vi "Check Path for Output.vi"(8 "error in (no error)":errorcluster, 10 "Path":path) -> (0 "error out":errorcluster)   [LabVIEW 2017, in "WebServiceImporter.lvlib" / "Main Panel.lvlib" / "Input Info.lvlib"]
uses:
  <vilib>/Platform/WebService/Main Panel/Pages/Input Info/Input Info.lvlib
  <vilib>/Platform/WebService/Error Handling/Error/Error Number.ctl
  <vilib>/Platform/WebService/Error Handling/Error Handling.lvlib
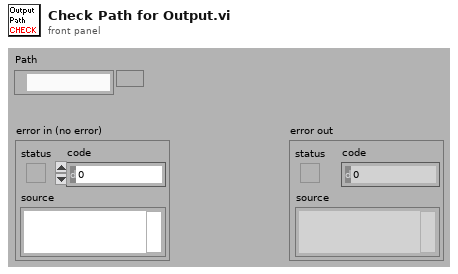
[diagram p1: front panel]
types:
  T1 = enum16{"open", "replace", "create", "open or create", "replace or create", "replace or create with confirmation"}
  T2 = typedef "WebServiceImporter.lvlib/Error Handling.lvlib/Error Number.ctl" = u16
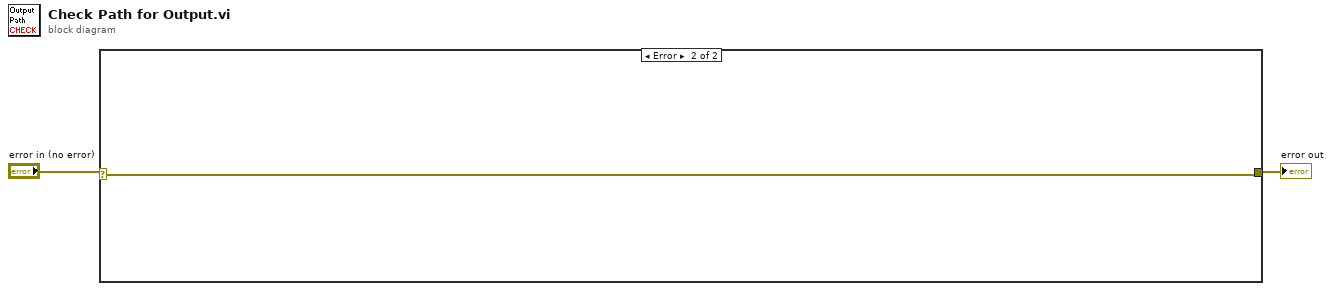
[diagram p0: block diagram]
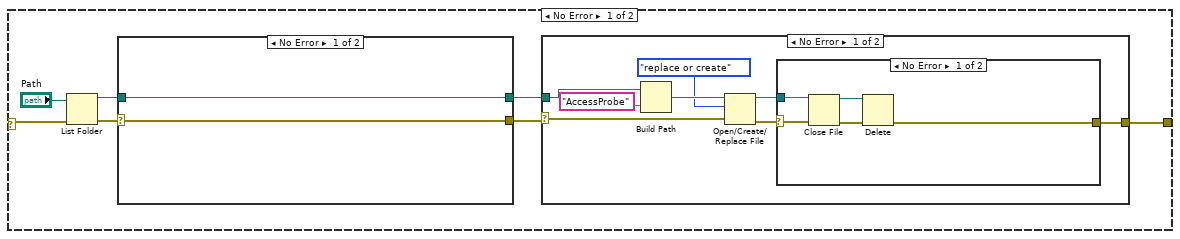
[diagram p2: hidden frame]
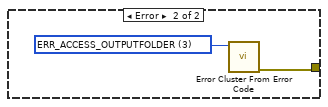
[diagram p3: hidden frame]
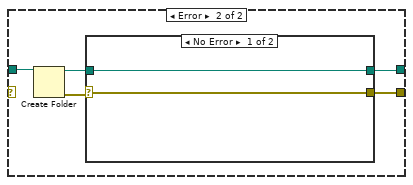
[diagram p5: hidden frame]
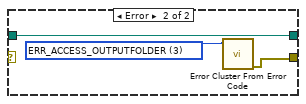
[diagram p6: hidden frame]
diagram:
  n1 = case shown="Error" "error in (no error)" {
    selector: "error in (no error)" -> [w3 w38]
    tunnel: [w5 w38] -> w2
    frame No Error {
      n2 = List Folder(path="Path", error in=w3) -> (path out=w8:path, error out=w7:errorcluster)  [unwired: 2 in, 2 out]
      n3 = case shown="No Error" w7 {
        selector: w7 -> [w27 _]
        tunnel: w8 -> [w26 w32]
        tunnel: [w27 w30] -> w6
        tunnel: [w26 w28] -> w4
        frame No Error {
        }
        frame Error {
          n4 = Create Folder(path (use dialog)=w32) -> (created path=w29:path, error out=w31:errorcluster)  [unwired: 2 in, 1 out]
          n5 = case shown="No Error" w31 {
            selector: w31 -> [w34 _]
            tunnel: [w34 w35] -> w30
            tunnel: w29 -> [w33 w37]
            tunnel: [w33 w37] -> w28
            frame No Error {
            }
            frame Error {
              w36 = T2 3 items=["No Error", "ERR_INVALID_WSDL", "ERR_CREATE_PROXYDLL", "ERR_ACCESS_OUTPUTFOLDER"] ("Error Number")
              n6 = call <vilib>:"Error Cluster From Error Code.vi"("error code (0)"=w36) -> ("error out"=w35:errorcluster)  [unwired: 8 in]
            }
          }
        }
      }
      n7 = case shown="No Error" w6 {
        selector: w6 -> [w13 w25]
        tunnel: [w10 w25] -> w5
        tunnel: w4 -> [w17 _]
        frame No Error {
          n8 = Build Path(base path=w17, name or relative path="AccessProbe") -> (appended path=w15:path)
          n9 = Open/Create/Replace File(file path (use dialog)=w15, error in=w13, operation (0:open)=T1."replace or create") -> (refnum out=w11:refnum<file>, error out=w12:errorcluster)  [unwired: 3 in, 1 out]
          n10 = case shown="No Error" w12 {
            selector: w12 -> [w22 _]
            tunnel: w11 -> [w21 _]
            tunnel: [w18 w23] -> w10
            frame No Error {
              n11 = Close File(refnum=w21, error in=w22) -> (path=w20:path, error out=w19:errorcluster)
              n12 = Delete(path (use dialog)=w20, error in=w19) -> (error out=w18:errorcluster)  [unwired: 3 in, 2 out]
            }
            frame Error {
              w24 = T2 3 items=["No Error", "ERR_INVALID_WSDL", "ERR_CREATE_PROXYDLL", "ERR_ACCESS_OUTPUTFOLDER"] ("Error Number")
              n13 = call <vilib>:"Error Cluster From Error Code.vi"("error code (0)"=w24) -> ("error out"=w23:errorcluster)  [unwired: 8 in]
            }
          }
        }
        frame Error {
        }
      }
    }
    frame Error {
    }
  }
  "error out" <- w2
